vi "PathPlanner_Segment_New.vi"(5 "P1":T5 {"Y" format="%14.3f"; "X" format="%14.3f"}, 6 "EndSegment":bool, 7 "P1 2":T5 {"Y" format="%14.3f"; "X" format="%14.3f"}, 8 "ConstraintZones":T1[](array[typedef]), 9 "TargetHolonomicRotations":T3[](array[typedef]) {"target"."SIN" format="%13.4f"; "target"."COS" format="%13.4f"; "target"."VALUE" format="%13.4f"}, 10 "P1 4":T5 {"Y" format="%14.3f"; "X" format="%14.3f"}, 11 "P1 3":T5 {"Y" format="%14.3f"; "X" format="%14.3f"}) -> (3 "Segment":T6 {"SegmentPoints"."HolonomicRotation"."SIN" format="%13.4f"; "SegmentPoints"."HolonomicRotation"."COS" format="%13.4f"; "SegmentPoints"."HolonomicRotation"."VALUE" format="%13.4f"; "SegmentPoints"."Position"."Y" format="%14.3f"; "SegmentPoints"."Position"."X" format="%14.3f"})   [LabVIEW 2019, in "PathPlanner24.lvlib"]
doc: "/**\n * Create a new path constraints object\n *\n * @param maxVelocityMps Max linear velocity (M/S)\n * @param maxAccelerationMpsSq Max linear acceleration (M/S^2)\n * @param maxAngularVelocityRps Max angular velocity (Rad/S)\n * @param maxAngularAccelerationRpsSq Max angular acceleration (Rad/S^2)\n */"
uses:
  PathPlanner24.lvlib
  TypeDef/PathPlannerPathConstraints.ctl
  <vilib>/Rock Robotics/WPI/ThirdParty/JAS_Junk/TrajLib/TypeDef/TRANSLATION2D.ctl
  <vilib>/Rock Robotics/WPI/ThirdParty/JAS_Junk/TrajLib/Trajectory_Library.lvlib
  <vilib>/Rock Robotics/WPI/ThirdParty/JAS_Junk/TrajLib/TypeDef/ROTATION2D.ctl
  TypeDef/PathPlannerPoint.ctl
  TypeDef/PathPlannerSegment.ctl
  TypeDef/PathPlannerRotationTarget.ctl
  TypeDef/PathPlannerConstraintsZone.ctl
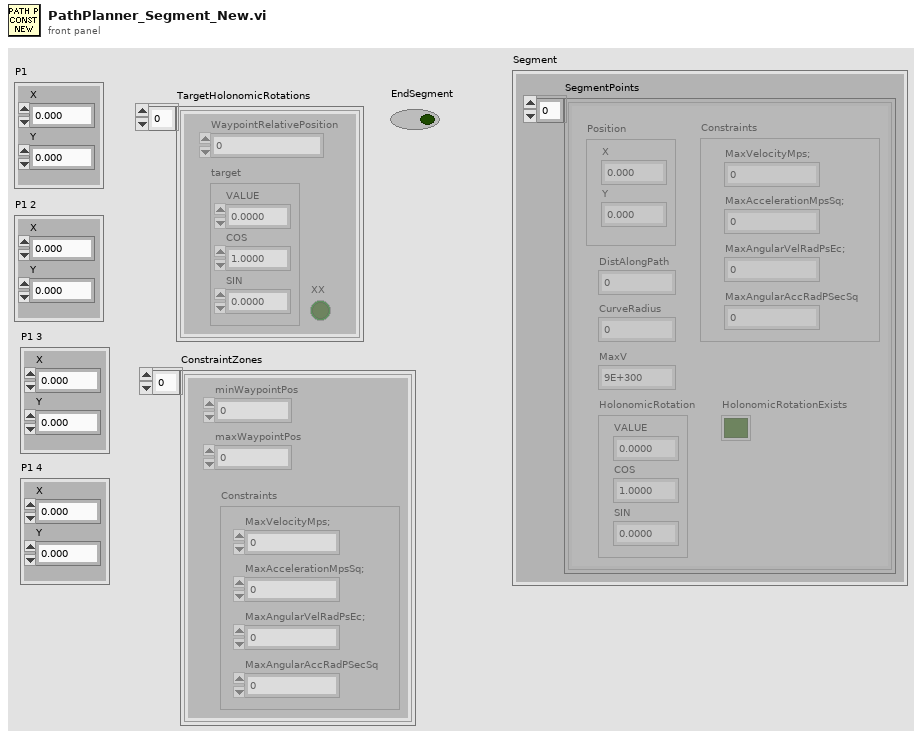
[diagram p1: front panel]
types:
  T1 = typedef "PathPlanner24.lvlib/PathPlannerConstraintsZone.ctl" = cluster{"minWaypointPos":dbl, "maxWaypointPos":dbl, "Constraints":T2}
  T2 = typedef "PathPlanner24.lvlib/PathPlannerPathConstraints.ctl" = cluster{"MaxVelocityMps;":dbl, "MaxAccelerationMpsSq;":dbl, "MaxAngularVelRadPsEc;":dbl, "MaxAngularAccRadPSecSq":dbl}
  T3 = typedef "PathPlanner24.lvlib/PathPlannerRotationTarget.ctl" = cluster{"target":T4, "WaypointRelativePosition":dbl, "XX":bool}
  T4 = typedef "Trajectory_Library.lvlib/ROTATION2D.ctl" = cluster{"VALUE":dbl, "COS":dbl, "SIN":dbl}
  T5 = typedef "Trajectory_Library.lvlib/TRANSLATION2D.ctl" = cluster{"X":dbl, "Y":dbl}
  T6 = typedef "PathPlanner24.lvlib/PathPlannerSegment.ctl" = cluster{"SegmentPoints":T7[]}
  T7 = typedef "PathPlanner24.lvlib/PathPlannerPoint.ctl" = cluster{"Position":T5, "HolonomicRotation":T4, "DistAlongPath":dbl, "CurveRadius":dbl, "MaxV":dbl, "Constraints":T2, "HolonomicRotationExists":bool}
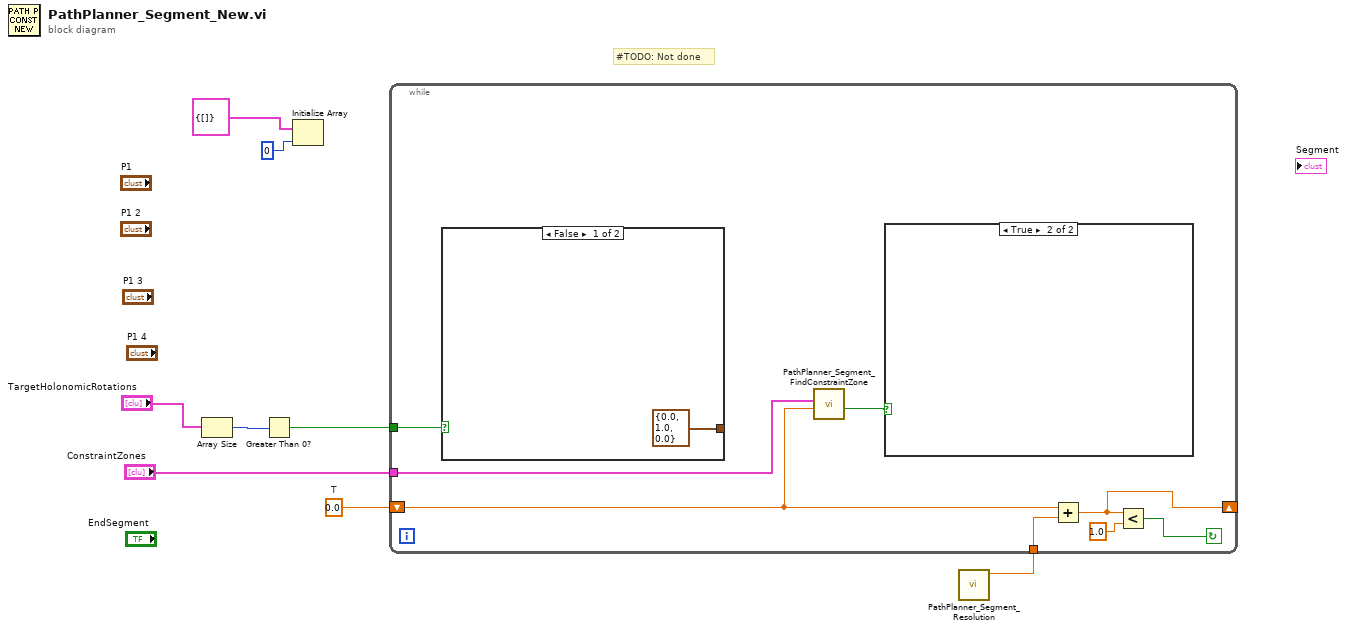
[diagram p0: block diagram]
diagram:
  w6 = 0.0  # T
  # "#TODO: Not done"
  n1 = Array Size(array="TargetHolonomicRotations") -> (size(s)=w3:i32)
  n2 = Greater Than 0?(x=w3) -> (x > 0?=w2:bool)
  n3 = Initialize Array(T6 {"SegmentPoints"=[]} ("Segment"), 0 ("dimension size")) -> ()  [unwired: 1 out]
  n4 = call "PathPlanner_Segment_Resolution.vi"() -> ("Resolution"=w5:dbl)  [unwired: 11 in]
  n5 = while {
    shift-right: [w14] -> _
    shift-left: w6 -> [w11]
    tunnel: w5 -> [w16]
    tunnel: w2 -> [w12]
    tunnel: "ConstraintZones" -> [w10]
    stop <- w13 continue-if-true
    n6 = case shown="False" w12 {
      tunnel: [T4 {"VALUE"=0.0, "COS"=1.0, "SIN"=0.0} ("ROTATION") _] -> _
      frame False {
      }
      frame True {
      }
    }
    n7 = call "PathPlanner_Segment_FindConstraintZone.vi"("T"=w11, "Zones"=w10) -> ("IsPresent"=w9:bool)  [unwired: 8 in, 1 out]
    n8 = case shown="True" w9 {
      frame False {
      }
      frame True {
      }
    }
    n9 = Add(x=w11, y=w16) -> (x+y=w14:dbl)
    n10 = Less?(x=w14, y=1.0) -> (x < y?=w13:bool)
  }
